vi "Script_Initialize Motor Communication.vi"(6 "error source terminal refnum":refnum<vi>, 7 "skip if name is empty (F)":bool, 8 "error in (no error)":errorcluster, 10 "owner diagram refnum":refnum<vi>, 11 "motor communication in":refnum<class "NI_Robotics_Motor Communication.lvclass">) -> (0 "error out":errorcluster, 1 "created?":bool, 2 "motor communication out terminal refnum":refnum<vi>, 3 "motor communication out":refnum<class "NI_Robotics_Motor Communication.lvclass">, 4 "error out terminal refnum":refnum<vi>)   [LabVIEW 2017, in "NI_Robotics_Scripting Utilities.lvlib"]
uses:
  <vilib>/robotics/Utilities/Scripting/NI_Robotics_Scripting Utilities.lvlib
  <vilib>/robotics/Actuation/Motor Communication/NI_Robotics_Motor Communication.lvclass
  <vilib>/robotics/Actuation/Motor Communication/NI_Robotics_Motor Communication.lvclass/NI_Robotics_Motor Communication.ctl
  <vilib>/Utility/miscctls.llb/LVPointTypeDef.ctl
  <vilib>/robotics/Actuation/Motor Communication/Initialize Motor Communication.vi
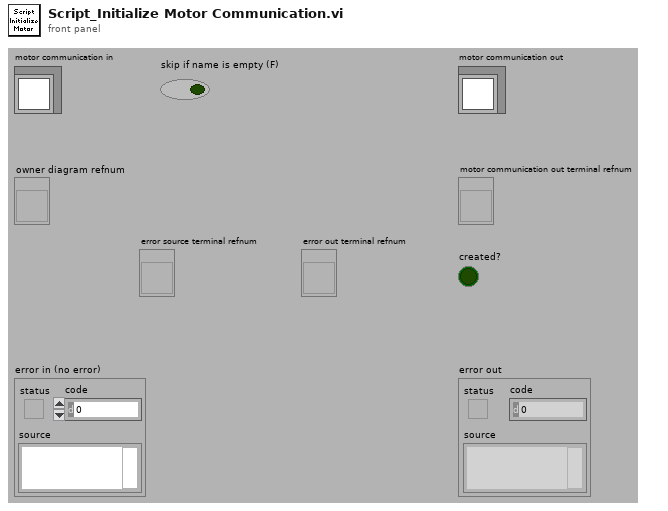
[diagram p1: front panel]
types:
  T1 = typedef "LVPointTypeDef.ctl" = cluster{"Horizontal":i16, "Vertical":i16}
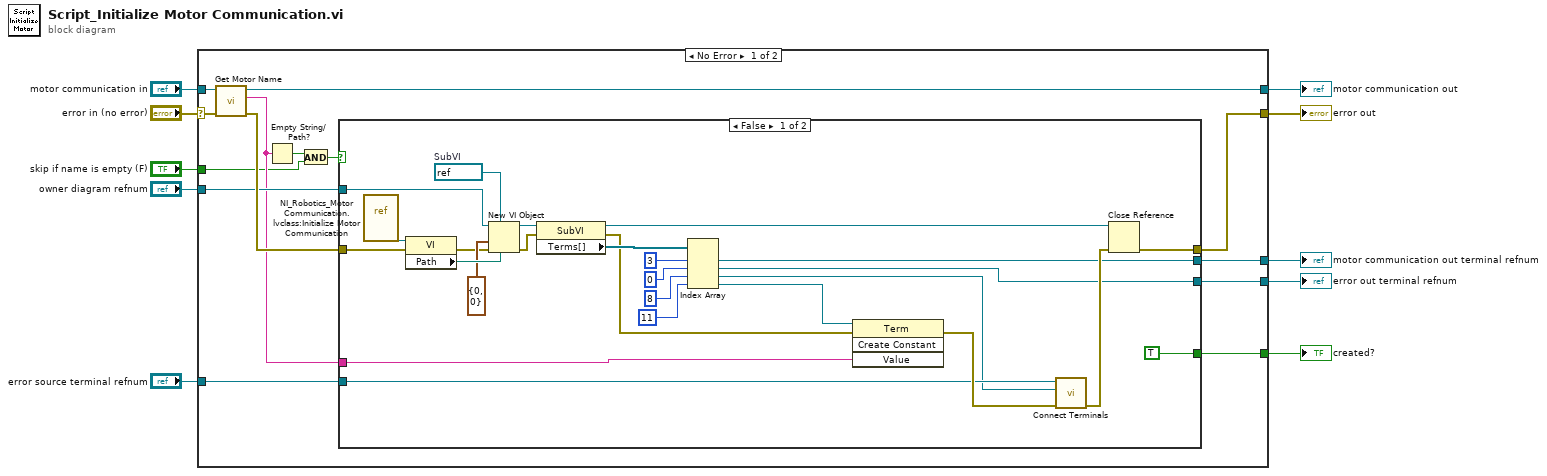
[diagram p0: block diagram]
diagram:
  n1 = case shown="No Error" "error in (no error)" {
    selector: "error in (no error)" -> [w22 w53]
    tunnel: [w19 w53] -> w9
    tunnel: [w23 w52] -> w7
    tunnel: "motor communication in" -> [w24 w52]
    tunnel: "owner diagram refnum" -> [w20 _]
    tunnel: [w18 _] -> w5
    tunnel: [w17 _] -> w4
    tunnel: "skip if name is empty (F)" -> [w14 _]
    tunnel: [w12 _] -> w2
    tunnel: "error source terminal refnum" -> [w11 _]
    frame No Error {
      n2 = call <vilib>:"Get Motor Name.vi"("error in (no error)"=w22, "motor communication in"=w24) -> ("error out"=w21:errorcluster, "motor name"=w16:string, "motor communication out"=w23:refnum<class "NI_Robotics_Motor Communication.lvclass">)  [unwired: 7 in]
      n3 = Empty String/Path?(string/path=w16) -> (empty?=w15:bool)
      n4 = And(x=w15, y=w14) -> (x .and. y?=w13:bool)
      n5 = case shown="False" w13 {
        tunnel: w21 -> [w44 w51]
        tunnel: w20 -> [w43 _]
        tunnel: [w42 w51] -> w19
        tunnel: [w27 _] -> w18
        tunnel: [w29 _] -> w17
        tunnel: w16 -> [w41 _]
        tunnel: [TRUE _] -> w12
        tunnel: w11 -> [w39 _]
        frame False {
          w48 = refnum<vi> refnum  # SubVI
          n6 = vi-ref "NI_Robotics_Motor Communication.lvclass:Initialize Motor Communication.vi"() -> (w49:refnum<vi>)
          n7 = property class="VI"(reference=w49, error in=w44) -> (error out=w46:errorcluster, "Path"=w50:path)  [unwired: 1 out]
          n8 = New VI Object(vi object class=w48, owner refnum=w43, position/next to=T1 {"Horizontal"=0, "Vertical"=0} ("relative position/next to refnum"), 6:w50, 8:w46) -> (object refnum=w37:refnum<vi>, 0:w26:errorcluster)  [unwired: 3 in]
          n9 = property class="SubVI"(reference=w37, error in=w26) -> (reference out=w36:refnum<vi>, error out=w25:errorcluster, "Terms[]"=w35:refnum<vi>[])
          n10 = Index Array(array=w35, index #1=3 ("index"), index #2=0 ("index"), index #3=8 ("index"), index #4=11 ("index")) -> (element #1=w29:refnum<vi>, element #2=w27:refnum<vi>, element #3=w31:refnum<vi>, element #4=w34:refnum<vi>)
          n11 = invoke class="Term" method="Create Constant"(reference=w34, error in=w25, "Value"=w41) -> (error out=w45:errorcluster)  [unwired: 1 in, 3 out]
          n12 = call <vilib>:"Connect Terminals.vi"("error in (no error)"=w45, "sink terminal"=w31, "source terminal"=w39) -> ("error out"=w38:errorcluster)  [unwired: 7 in, 1 out]
          n13 = Close Reference(reference=w36, error in (no error)=w38) -> (error out=w42:errorcluster)
        }
        frame True {
        }
      }
    }
    frame Error {
    }
  }
  "error out" <- w9
  "motor communication out" <- w7
  "motor communication out terminal refnum" <- w4
  "error out terminal refnum" <- w5
  "created?" <- w2
